vi "bit_True_False.vi"(5 "number":u32) -> (2 "True?":bool)   [LabVIEW 2021]
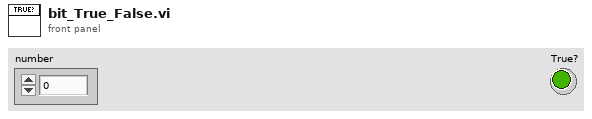
[diagram p1: front panel]
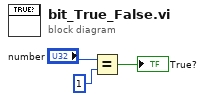
[diagram p0: block diagram]
diagram:
  n1 = Equal?(x="number", y=u32 1) -> (x = y?=→"True?":bool)
